vi "CIPT_softwarecontrol with touching pins.vi"() -> ()   [LabVIEW 2022 SP3]
uses:
  Git/CIPT/CIPT/Labview Project/CIPT modes.ctl
  <vilib>/Analysis/baseanly.llb/Mean (DBL).vi
  <vilib>/Utility/file.llb/Read Delimited Spreadsheet (DBL).vi
  <vilib>/Utility/file.llb/Read Delimited Spreadsheet (I64).vi
  <vilib>/gmath/NumericalOptimization/Nonlinear Curve Fit LM.vi
  <vilib>/Utility/file.llb/Write Delimited Spreadsheet (string).vi
  <vilib>/Utility/file.llb/Write Delimited Spreadsheet (I64).vi
  <vilib>/Utility/file.llb/Write Delimited Spreadsheet (DBL).vi
  C:/CIPT/Labview Project/Camera Driver/Labview Driver/OtherDrivers/LabVIEW/ueye.NET/uEyeDotNet.dll
  CIPT/Labview Project/Camera Driver/Labview Driver/OtherDrivers/LabVIEW/ueye.NET/uEyeDotNet.dll
  <vilib>/gmath/NI_Gmath.lvlib
  <instrlib>/Keithley DMM6500 DAQ6500 Series/Keithley DMM6500 DAQ6500 Series.lvlib
  <instrlib>/Keithley 24XX/Keithley 24XX.lvlib
  <instrlib>/Keithley 2182/Keithley 2182.lvlib
  <vilib>/Analysis/NI_AALBase.lvlib
panel:
  out "Array":dbl[](array[numeric])
  out "Comms Errors":errorcluster[](array[cluster])
  in  "Save Filr":bool
  out "error file out":errorcluster
  in  "output file path":path=path "C:/CIPT/Labview Project/csv files/test output.csv"
  in  "stop":bool
  in  "Tab Control":T1(tab)
  in  "Camera ID 3":enum16{"2", "1"}(ring)
  in  "Camera ID 1":enum16{"2", "1"}(ring)
  in  "down a2":bool
  in  "up a2":bool
  in  "down a1":bool
  in  "up a1":bool
  in  "down a3":bool
  in  "up a3":bool
  in  "down all":bool
  in  "up all":bool
  in  "steps /\n continuous \ntoggle":bool
  out "Image first camera":picture
  out "Serial Number 1":string
  in  "Init Camera":bool
  in  "Exit Camera":bool
  in  "Init Camera 2":bool
  in  "Exit Camera 2":bool
  out "Serial Number 2":string
  out "Image second camera":picture
  out "Error Camera 1":errorcluster caption="error"
  out "Error Camera 2":errorcluster caption="error"
  in  "COM 1":refnum<visa-resource-name>
  out "error":errorcluster
  in  "Probe Landing File":path=path "C:/CIPT/Labview Project/csv files/Probe Landing cipt.csv"
  in  "Landing Test on/off?":bool
  in  "load file":bool
  in  "Step size":i32=10
  out "Measurement":sgl[](array[numeric])
  out "Loaded":bool
  out "Loaded":bool
  out "Error Probe Configuration File":errorcluster
  in  "Probe Configuration File":path=path "C:/CIPT/Labview Project/csv files/test probe config.csv"
  in  "Probe Settings File":path=path "C:/CIPT/Labview Project/csv files/deafult_probe_setrings.CSV"
  out "Error Probe Settings File":errorcluster
  out "Probe Spacings":dbl[][](array[numeric])
  in  "Load":bool
  in  "Multiplexer":refnum<visa-resource-name>
  out "all rows":i64[][](array[numeric])
  out "Results Description":string[](array[string])
  out "Results":dbl[][](array[numeric])
  out "Probe Set 2":i32
  in  "Compliance voltage (V)":dbl=42.0
  in  "Measure Instrument":refnum<visa-resource-name>
  in  "Radio Buttons":T2 caption="Select Instrumentation"
  in  "Source Instrument":refnum<visa-resource-name>
  in  "Run":bool
  in  "Current (µA)":dbl=10.0
  out "Measurement Log":string
  out "Probe Set":i32
  in  "Measurement Repeats":i32=10
  in  "Size Of Buffer Used For One Measurement":i32=3
  in  "Top Film R est.":dbl=0.25
  in  "Bottm Film R est.":dbl=0.25
  in  "RA est.":dbl=0.25
  out "Top Film R":dbl
  out "Bottom Film R":dbl
  out "RA":dbl
  out "error out (fitting model)":errorcluster
  in  "Fit Data":bool
  out "Measurements Map Out":map{string, dbl[]}(c390)
  # "Probe Landing cipt_probe check: checks probes individually \nProbe Landing cipt: checks for any connection"
  # "All"
  # "End"
  # "home"
  # "Delete"
  # "Insert"
  # "Page Down"
  # "Page up"
  # "F2"
  # "F1"
  # "Steps"
  # "Continuous"
  # "Probe Settings"
  # "Probe Configuration"
  # "I+"
  # "V+"
  # "V-"
  # "I-"
  # "Max Resolution of 2400 is 300 µV in 200 mV range"
  # "/"
  # "Sheet Resistance (RA)"
  # "Estimated Values"
  # "Fitted Values"
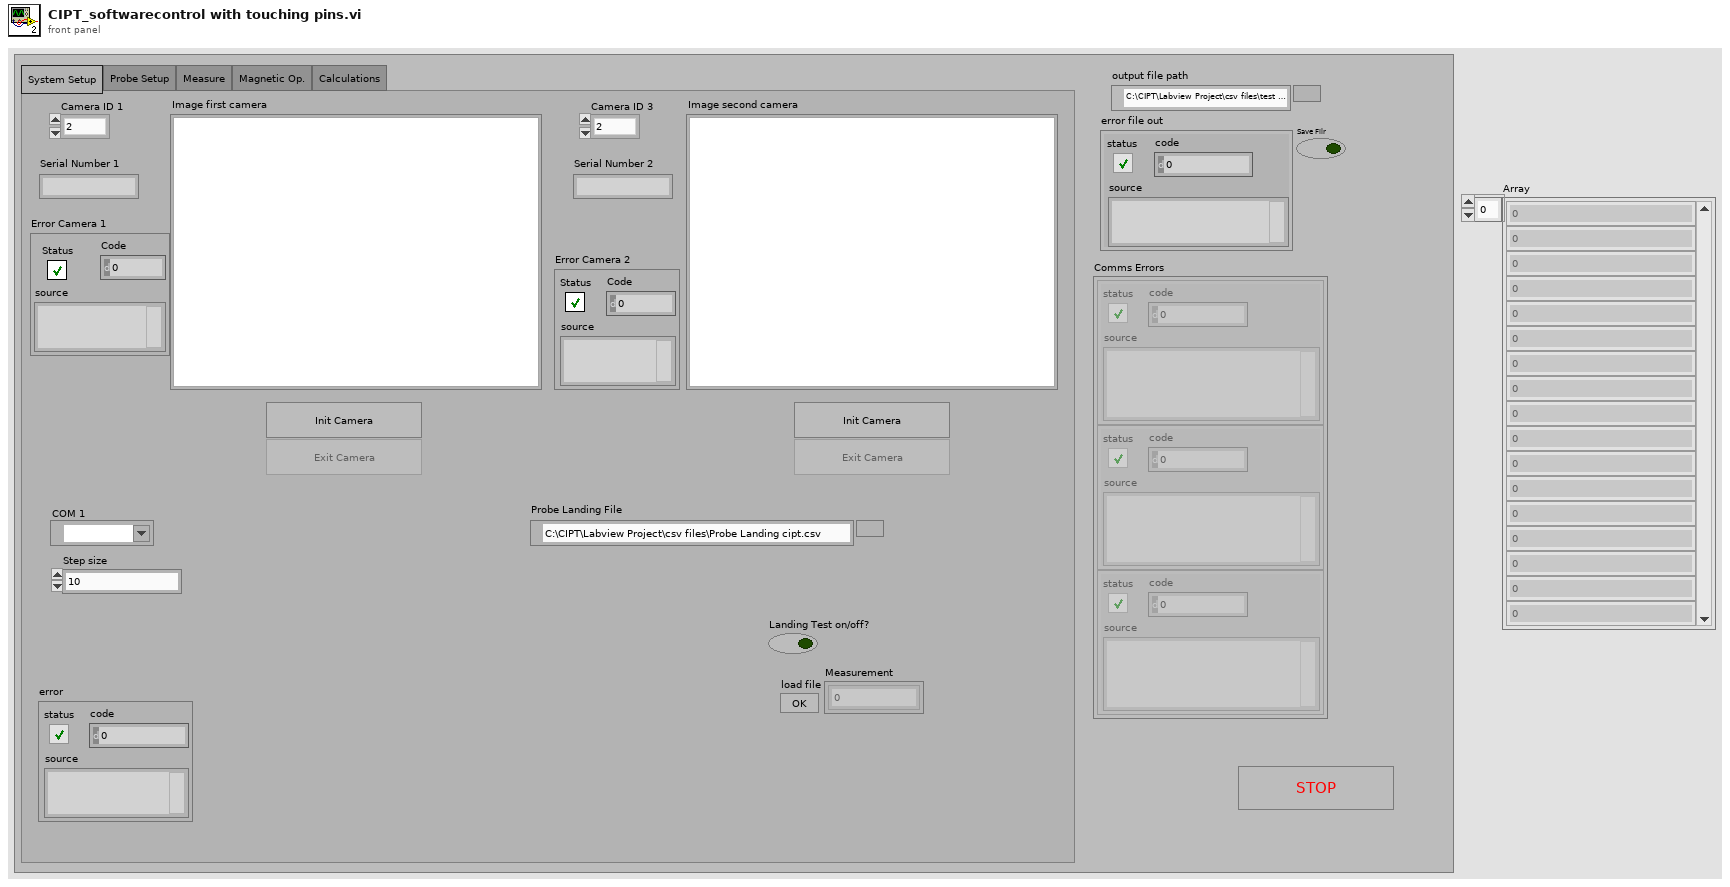
[diagram p1: front panel]
types:
  T1 = enum32{"System Setup", "Probe Setup", "Measure", "Magnetic Op.", "Calculations"}
  T2 = typedef "CIPT modes.ctl" = enum32{"DAQ6510", "2400 Only", "2400 and  2182", "SR830", "SR830 and 6221"}
  T3 = enum32{"System Setup", "Probe Setup", "Measure", "Magnetic Operations", "Calculations + Analyis"}
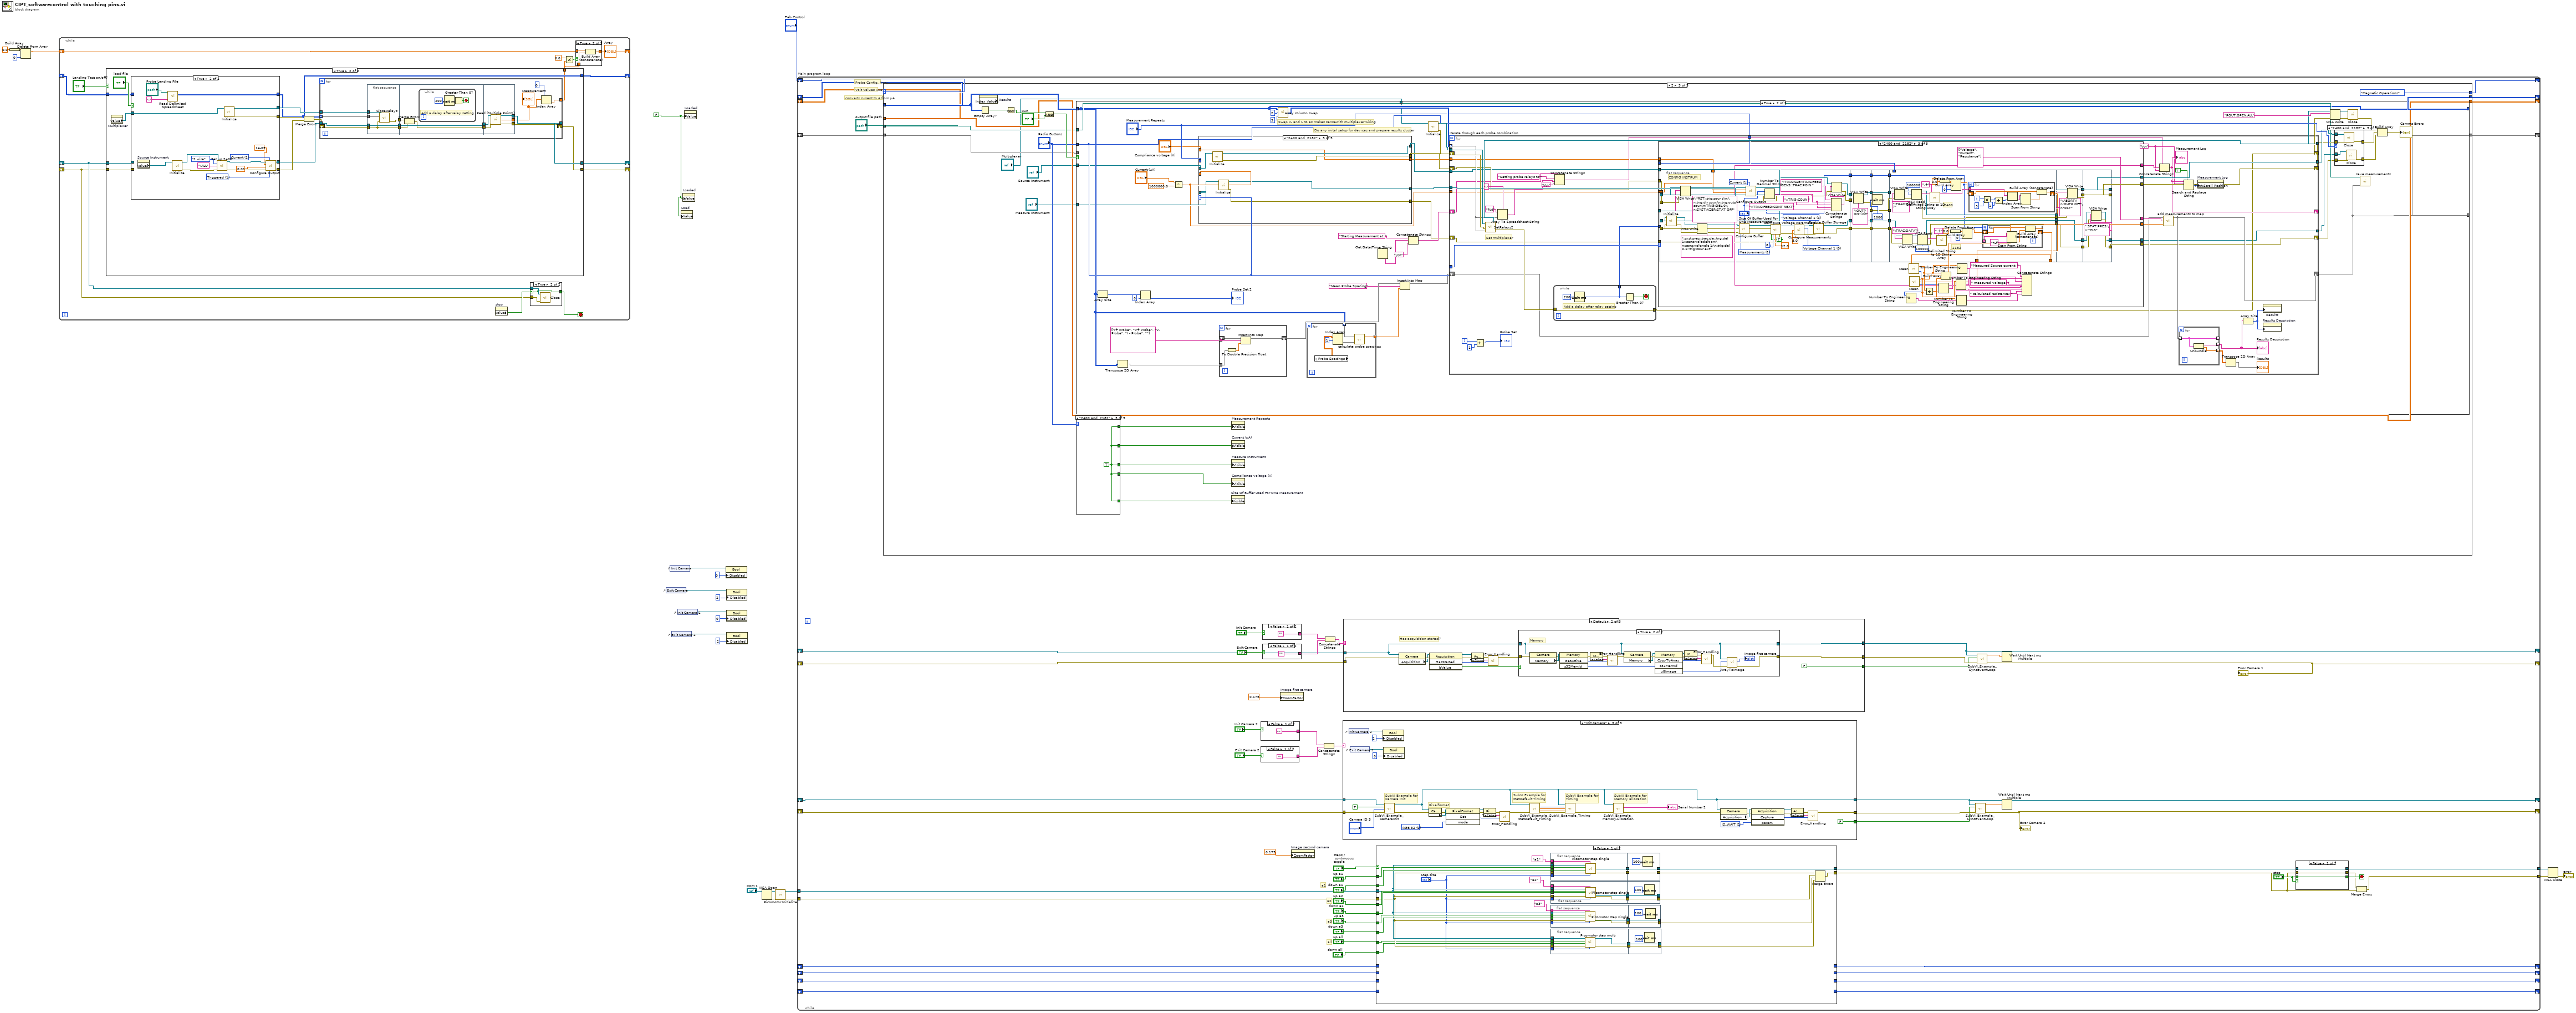
[diagram p0: block diagram]
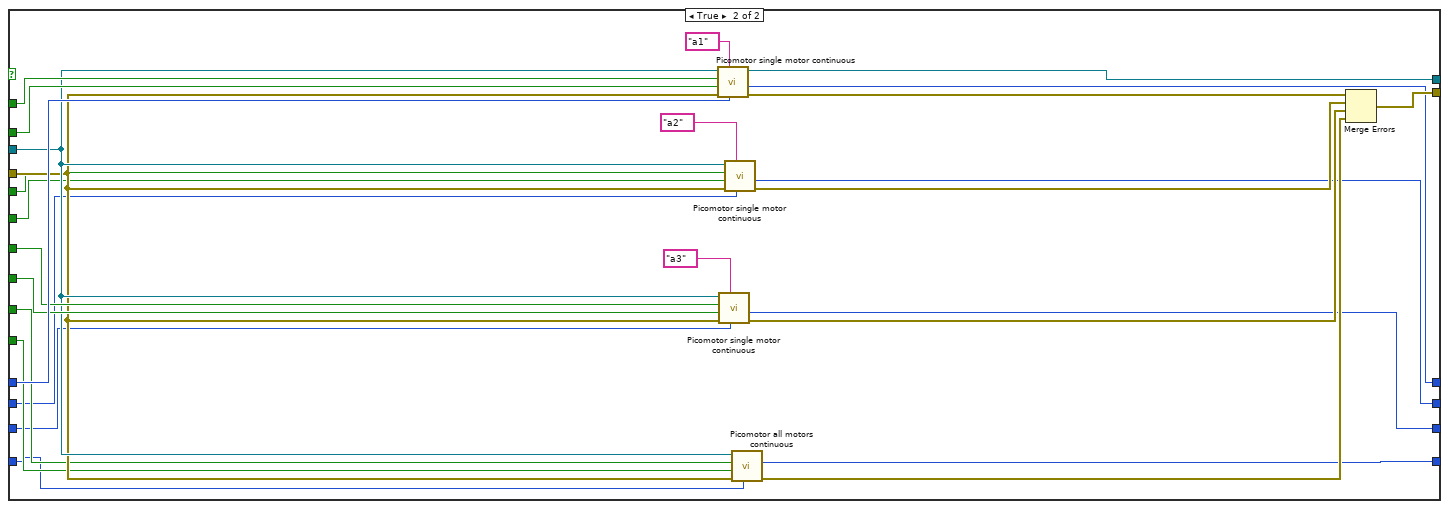
[diagram p6: hidden frame]
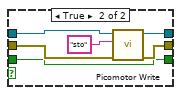
[diagram p7: hidden frame]
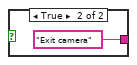
[diagram p8: hidden frame]
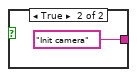
[diagram p9: hidden frame]
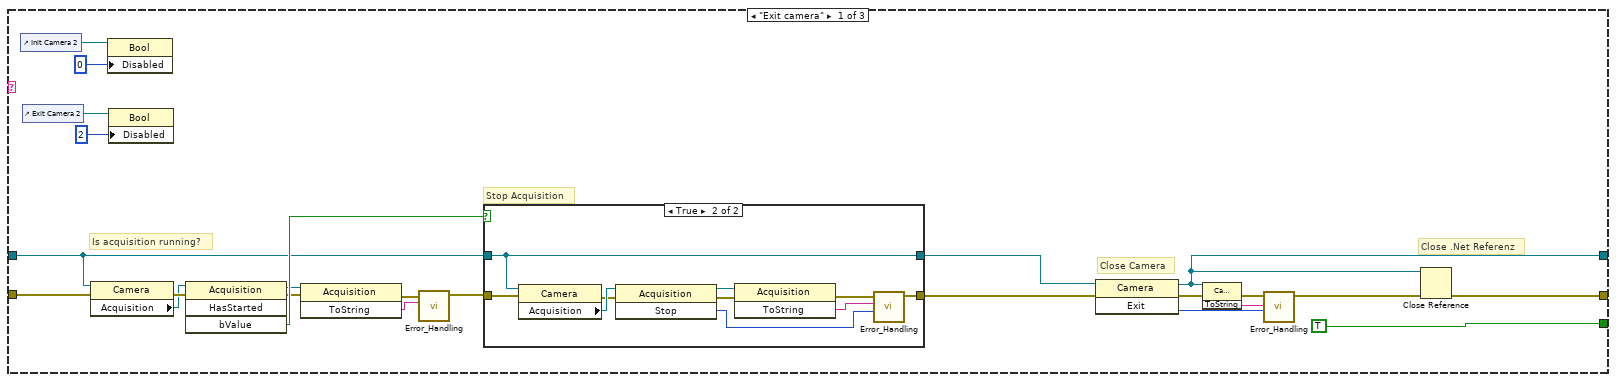
[diagram p10: hidden frame]
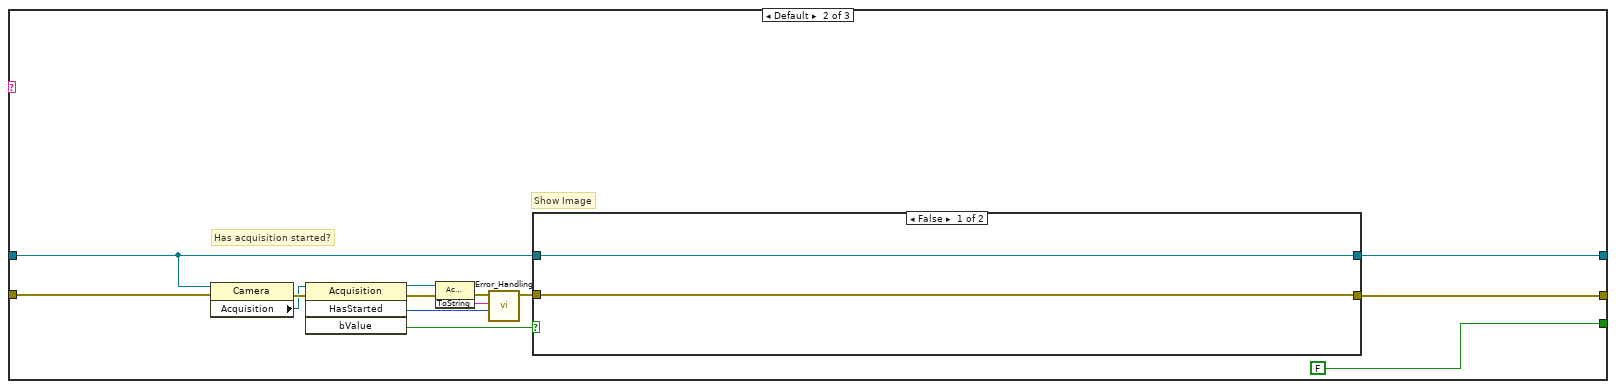
[diagram p12: hidden frame]
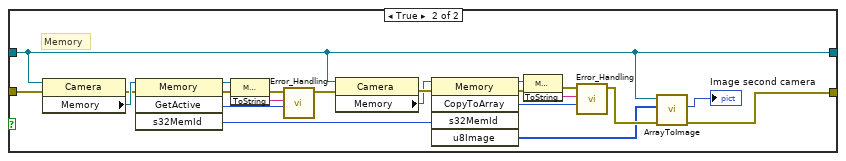
[diagram p13: hidden frame]
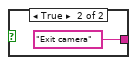
[diagram p14: hidden frame]
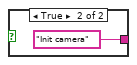
[diagram p15: hidden frame]
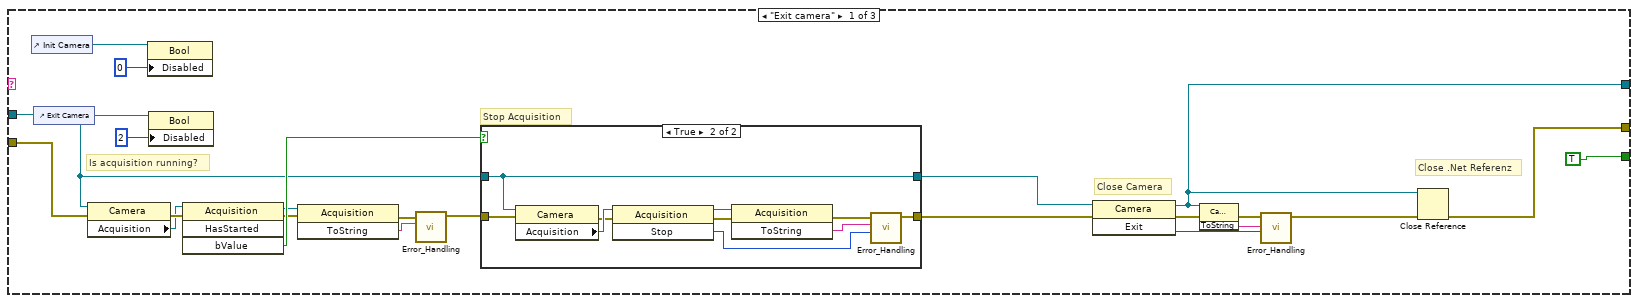
[diagram p16: hidden frame]
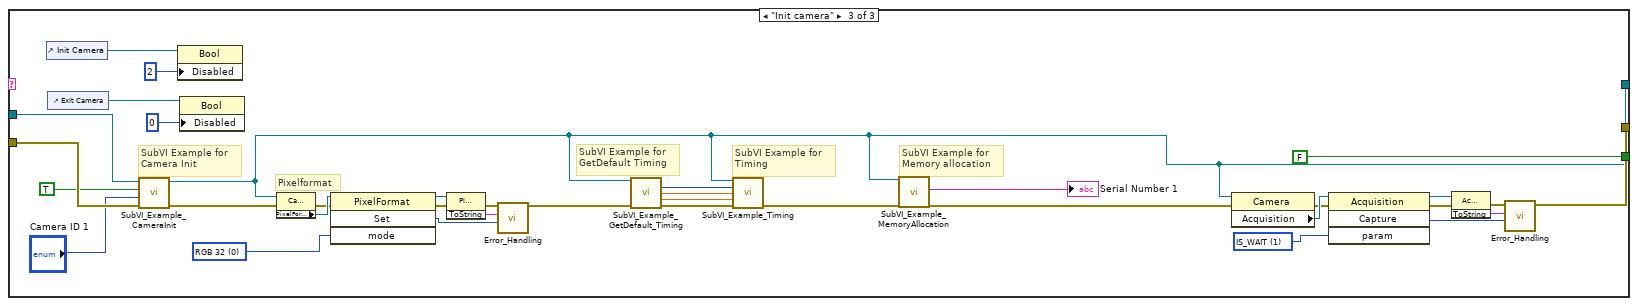
[diagram p19: hidden frame]
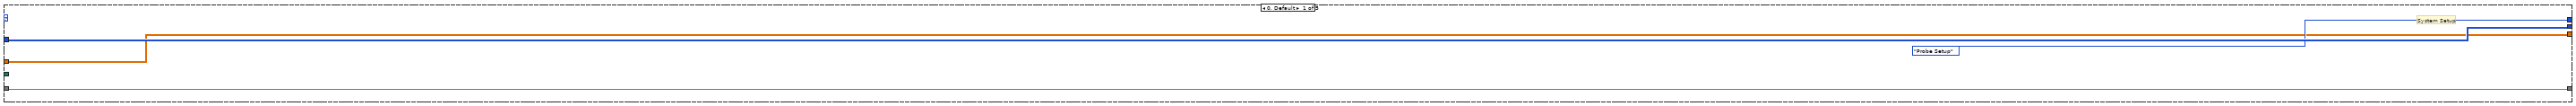
[diagram p20: hidden frame]
diagram:
  w13 = FALSE
  n1 = Build Array(0.0 ("array")) -> (w3:dbl[])
  n2 = Delete From Array(array=w3, index=0) -> (array with subset deleted=w1:dbl[])  [unwired: 1 in, 1 out]
  n3 = while {
    shift-right: [w35] -> _
    shift-left: _ -> [w32]
    shift-right: [w34] -> _
    shift-left: _ -> [w31]
    shift-right: [w29] -> _
    shift-left: _ -> [w28]
    shift-right: [w27] -> _
    shift-left: w1 -> [w26]
    stop <- w30 stop-if-true
    n4 = case shown="True" "Landing Test on/off?" {
      tunnel: w32 -> [w47 w56]
      tunnel: w31 -> [w46 w55]
      tunnel: [w47 w54] -> w35
      tunnel: [w46 w53] -> w34
      tunnel: w28 -> [w45 w50]
      tunnel: [w45 w49] -> w29
      tunnel: [_ w48] -> w24
      frame False {
      }
      frame True {
        n5 = property on="Multiplexer" class="VISAName"() -> ("Value"=w52:refnum<visa-resource-name>)  [unwired: 2 in, 2 out]
        n6 = case shown="True" "load file" {
          tunnel: [_ w99] -> w61
          tunnel: [w95 w102] -> w58
          tunnel: [w96 w101] -> w57
          tunnel: w56 -> [w96 _]
          tunnel: w55 -> [w95 _]
          tunnel: [w94 w100] -> w51
          tunnel: w52 -> [w94 w98]
          tunnel: [w93 w97] -> w49
          tunnel: w50 -> [w93 _]
          frame False {
          }
          frame True {
            w108 = u16 1 items=["Immediate", "Triggered"] ("Output Type  (0: Immediate)")
            w107 = u16 1 items=["Voltage", "Current"] ("Source Mode  (0: Voltage)")
            n7 = property on="Source Instrument" class="VISAName"() -> ("Value"=w113:refnum<visa-resource-name>)  [unwired: 2 in, 2 out]
            n8 = call-poly <vilib>:"Read Delimited Spreadsheet.vi"("file path (dialog if empty)"="Probe Landing File", "delimiter (\\t)"="," ("delimiter (\\t)")) -> ("all rows"=w97:i64[][])  [unwired: 8 in, 5 out]
            n9 = call <instrlib>:"Initialize.vi"("VISA resource name"=w113) -> ("error out"=w110:errorcluster, "VISA resource name out"=w109:refnum<visa-resource-name>)  [unwired: 9 in]
            n10 = call "Set up 2400.vi"("VISA resource name"=w109, "Sense mode"=enum16{"2 wire", "4 wire"}."2 wire", "Measurement Function"=":ALL", "error in (no error)"=w110) -> ("VISA resource name out"=w111:refnum<visa-resource-name>, "error out"=w112:errorcluster)  [unwired: 10 in]
            n11 = call <instrlib>:"Initialize.vi"("VISA resource name"=w98) -> ("error out"=w99:errorcluster, "VISA resource name out"=w100:refnum<visa-resource-name>)  [unwired: 9 in]
            n12 = call <instrlib>:"Configure Output.vi"("Output Type  (0: Immediate)"=w108, "Source Mode  (0: Voltage)"=w107, "error in (no error)"=w112, "Compliance  Level (0.1)"=0.01, "Output Level (0)"=1e-05, "VISA resource name"=w111) -> ("error out"=w102:errorcluster, "VISA resource name out"=w101:refnum<visa-resource-name>)  [unwired: 4 in]
          }
        }
        n13 = Merge Errors(w61, w58) -> (w60:errorcluster)
        n14 = for {
          tunnel: w51 -> [w66]
          shift-right: [w67] -> w53
          shift-left: w60 -> [w70]
          tunnel: w49 -> [w65] mode=indexing
          tunnel: w57 -> [w69]
          tunnel: [w68] -> w54
          tunnel: [w62] -> w48
          n15 = flat-sequence {
            tunnel: w69 -> [w80]
            tunnel: w70 -> [w76]
            tunnel: [w76] -> w75
            tunnel: [w80] -> w74
            tunnel: w66 -> [w79]
            tunnel: [w78] -> w73
            tunnel: w65 -> [w77]
            tunnel: [w82] -> w72
            tunnel: [w84] -> w71
            tunnel: w75 -> [w83]
            tunnel: w74 -> [w84]
            tunnel: w73 -> [w81]
            tunnel: [w90] -> w64
            tunnel: [w89] -> w68
            tunnel: [w88] -> w67
            tunnel: w72 -> [w92]
            tunnel: w71 -> [w91]
            frame #0 {
              n16 = call "CloseRelays.vi"("error in (no error)"=w76, "Array"=w77, "VISA Refnum in"=w79) -> ("error out"=w78:errorcluster)  [unwired: 6 in, 2 out]
            }
            frame #1 {
              n17 = Merge Errors(w81, w83) -> (w82:errorcluster)
              n18 = while {
                stop <- w86 stop-if-true
                # "Add a delay after relay setting"
                n19 = Wait (ms)(milliseconds to wait=u32 200) -> (millisecond timer value=w85:u32)
                n20 = Greater Than 0?(x=w85) -> (x > 0?=w86:bool)
              }
            }
            frame #2 {
              n21 = call <instrlib>:"Read (Multiple Points).vi"("VISA resource name"=w91, "error in (no error)"=w92) -> ("VISA resource name out"=w89:refnum<visa-resource-name>, "Resistance"=w90:sgl[], "error out"=w88:errorcluster)  [unwired: 7 in, 4 out]
            }
          }
          n22 = Index Array(array=w64, index=0) -> (element=w62:sgl)
          "Measurement" <- w64
        }
      }
    }
    n23 = property on="stop" class="Bool (strict)"() -> ("Value"=w33:bool)  [unwired: 2 in, 2 out]
    n24 = case shown="True" w33 {
      selector: w33 -> [w41 w42]
      tunnel: w32 -> [_ w44]
      tunnel: w31 -> [_ w43]
      tunnel: [w41 w42] -> w30
      frame False {
      }
      frame True {
        n25 = call <instrlib>:"Close.vi"("error in (no error)"=w43, "VISA resource name"=w44) -> ()  [unwired: 9 in, 1 out]
      }
    }
    n26 = Not Equal?(x=sgl 0.0, y=w24) -> (x != y?=w25:bool)
    n27 = case shown="True" w25 {
      tunnel: w24 -> [_ w40]
      tunnel: [w37 w39] -> w27
      tunnel: w26 -> [w37 w38]
      frame False {
      }
      frame True {
        n28 = Build Array (concatenate)(w38, w40) -> (w39:dbl[])
      }
    }
    "Array" <- w27
  }
  n29 = control-ref of="Exit Camera"() -> (w16:refnum<vi>)
  n30 = control-ref of="Init Camera"() -> (w17:refnum<vi>)
  n31 = control-ref of="Exit Camera 2"() -> (w21:refnum<vi>)
  n32 = control-ref of="Init Camera 2"() -> (w20:refnum<vi>)
  n33 = property on="Load" class="Bool (strict)"("Value"=w13) -> ()  [unwired: 2 in, 2 out]
  n34 = property on="Loaded" class="Bool (strict)"("Value"=w13) -> ()  [unwired: 2 in, 2 out]
  n35 = property on="Loaded" class="Bool (strict)"("Value"=w13) -> ()  [unwired: 2 in, 2 out]
  n36 = property class="Bool"(reference=w17, "Disabled"=u8 0 ("Deaktiviert")) -> ()  [unwired: 1 in, 2 out]
  n37 = property class="Bool"(reference=w16, "Disabled"=u8 2 ("Deaktiviert")) -> ()  [unwired: 1 in, 2 out]
  n38 = property class="Bool"(reference=w20, "Disabled"=u8 0 ("Deaktiviert")) -> ()  [unwired: 1 in, 2 out]
  n39 = property class="Bool"(reference=w21, "Disabled"=u8 2 ("Deaktiviert")) -> ()  [unwired: 1 in, 2 out]
  n40 = VISA Open(VISA resource name="COM 1") -> (VISA resource name=w11:refnum<visa-resource-name>, error out=w10:errorcluster)  [unwired: 4 in]
  n41 = call "Picomotor Initialize.vi"("error in (no error)"=w10, "VISA Refnum in"=w11) -> ("error out"=w8:errorcluster, "VISA Refnum out"=w9:refnum<visa-resource-name>)  [unwired: 8 in]
  n42 = while "Main program loop" {
    shift-right: [w174] -> _
    shift-left: _ -> [w175]
    shift-right: [w173] -> _
    shift-left: "Tab Control" -> [w176]
    shift-right: [w172] -> _
    shift-left: _ -> [w171]
    shift-right: [w169] -> _
    shift-left: _ -> [w168]
    shift-right: [w157] -> _
    shift-left: _ -> [w155]
    shift-right: [w158] -> _
    shift-left: _ -> [w156]
    shift-right: [w145] -> _
    shift-left: _ -> [w143]
    shift-right: [w144] -> _
    shift-left: _ -> [w142]
    tunnel: w9 -> [w129]
    tunnel: w8 -> [w128]
    tunnel: [w141] -> w6
    shift-right: [w126] -> _
    shift-left: _ -> [w122]
    shift-right: [w125] -> _
    shift-left: _ -> [w121]
    shift-right: [w124] -> _
    shift-left: _ -> [w120]
    shift-right: [w123] -> _
    shift-left: _ -> [w119]
    tunnel: [w116] -> w5
    stop <- w140 stop-if-true
    # "a2"
    # "a3"
    # "all"
    # "a1"
    # "converts current to A from µA"
    # "Volt Values Array"
    # "Probe Config. Array"
    n43 = case shown="2" w176 {
      tunnel: w175 -> [w515 w522 w552 w911 w918]
      tunnel: [w515 w526 w551 w911 w918] -> w174
      tunnel: [T3."Probe Setup" ("Tab Control") T3."Measure" ("Tab Control") T3."Magnetic Operations" ("Tab Control") T3."Calculations + Analyis" ("Tab Control") T3."System Setup" ("Tab Control")] -> w173
      tunnel: [w513 w521 w546 w910 w917] -> w172
      tunnel: w171 -> [w513 w520 w546 w910 w917]
      tunnel: "output file path" -> [_ _ w543 _ w916]
      tunnel: [w512 w517 w542 w909 w915] -> w169
      tunnel: w168 -> [w512 w517 w541 w909 w915]
      frame 0, Default {
        # "System Setup"
      }
      frame 1 {
        # "Probe Setup"
        n44 = Empty Array?(array=w522) -> (empty?=w516:bool)
        n45 = Empty Array?(array=w520) -> (empty?=w519:bool)
        n46 = Not(x=w516) -> (.not. x?=→"Loaded":bool)
        n47 = Not(x=w519) -> (.not. x?=→"Loaded":bool)
        n48 = case shown="True" "Load" {
          tunnel: [w528 w529] -> w526
          tunnel: w522 -> [w528 _]
          tunnel: [w527 w530] -> w521
          tunnel: w520 -> [w527 _]
          frame False {
          }
          frame True {
            # "Probe config. file and data aquisition"
            # "Probe settings file and data aquisition"
            n49 = call-poly <vilib>:"Read Delimited Spreadsheet.vi"("file path (dialog if empty)"="Probe Configuration File", "delimiter (\\t)"="," ("delimiter (\\t)")) -> ("all rows"=w529:i64[][], "error out"=→"Error Probe Configuration File":errorcluster)  [unwired: 8 in, 4 out]
            "all rows" <- w529
            n50 = call-poly <vilib>:"Read Delimited Spreadsheet.vi"("file path (dialog if empty)"="Probe Settings File", "delimiter (\\t)"="," ("delimiter (\\t)")) -> ("all rows"=w530:dbl[][], "error out"=→"Error Probe Settings File":errorcluster)  [unwired: 8 in, 4 out]
            "Probe Spacings" <- w530
          }
        }
        n51 = property on="Load" class="Bool (strict)"("Value"=w516) -> ()  [unwired: 2 in, 2 out]
      }
      frame 2 {
        n52 = property on="Results" class="Arr (strict)" props=["Index Values"]() -> ()  [unwired: 2 in, 3 out]
        n53 = Empty Array?(array=w552) -> (empty?=w554:bool)
        n54 = Not(x=w554) -> (.not. x?=w553:bool)
        n55 = Compound Arithmetic op=AND(w553, "Run") -> (w556:bool)
        n56 = case shown="True" w556 {
          tunnel: w552 -> [w567 w586]
          tunnel: [w567 w586] -> w551
          tunnel: "Radio Buttons" -> [_ w612]
          tunnel: w543 -> [_ w600]
          tunnel: [w566 w582] -> w542
          tunnel: w541 -> [w566 _]
          tunnel: "Measure Instrument" -> [_ w574]
          tunnel: "Source Instrument" -> [_ w573]
          tunnel: "Multiplexer" -> [_ w572]
          frame False {
          }
          frame True {
            # "Swap V- and I- to as makes sensewith multiplexer wiring"
            # "Do any inital setup for devices and prepare results cluster"
            n57 = Array Size(array=w586) -> (size(s)=w606:i32[])
            n58 = Transpose 2D Array(2D array=w586) -> (transposed array=w585:i64[][])
            n59 = Index Array "Index Array"(array=w606, index=0) -> (element=→"Probe Set 2":i32)
            n60 = Divide(x="Current (µA)", y=1000000.0) -> (x/y=w568:dbl)
            n61 = case shown="\"2400 and  2182\"" w612 {
              tunnel: w573 -> [_ w650 w656 _ _]
              tunnel: [_ w638 w655 _ _] -> w613
              tunnel: w574 -> [_ _ w657 _ _]
              tunnel: [_ w638 w653 _ _] -> w576
              tunnel: [_ w644 w652 _ _] -> w607
              tunnel: w568 -> [_ w641 _ _ _]
              tunnel: "Compliance voltage (V)" -> [_ w639 w651 _ _]
              tunnel: "Measurement Repeats" -> [_ _ _ _ _]
              tunnel: [_ _ w654 _ _] -> w571
              tunnel: [_ _ w651 _ _] -> w569
              frame "DAQ6510", Default {
              }
              frame "2400 Only" {
                w642 = u16 1 items=["Immediate", "Triggered"] ("Output Type  (0: Immediate)")
                w643 = u16 1 items=["Voltage", "Current"] ("Source Mode  (0: Voltage)")
                n62 = call <instrlib>:"Initialize.vi"("VISA resource name"=w650) -> ("error out"=w648:errorcluster, "VISA resource name out"=w649:refnum<visa-resource-name>)  [unwired: 9 in]
                n63 = call "Set up 2400.vi"("VISA resource name"=w649, "Sense mode"=enum16{"2 wire", "4 wire"}."4 wire", "Measurement Function"=":ALL", "error in (no error)"=w648) -> ("VISA resource name out"=w646:refnum<visa-resource-name>, "error out"=w645:errorcluster)  [unwired: 10 in]
                n64 = call <instrlib>:"Configure Output.vi"("Output Type  (0: Immediate)"=w642, "Source Mode  (0: Voltage)"=w643, "error in (no error)"=w645, "Compliance  Level (0.1)"=w639, "Output Level (0)"=w641, "VISA resource name"=w646) -> ("error out"=w644:errorcluster, "VISA resource name out"=w638:refnum<visa-resource-name>)  [unwired: 4 in]
              }
              frame "2400 and  2182" {
                n65 = call <instrlib>:"Initialize.vi"("VISA resource name"=w656) -> ("error out"=w652:errorcluster, "VISA resource name out"=w653:refnum<visa-resource-name>)  [unwired: 9 in]
                n66 = call <instrlib>:"Initialize.vi"("VISA resource name"=w657) -> ("error out"=w654:errorcluster, "VISA resource name out"=w655:refnum<visa-resource-name>)  [unwired: 9 in]
              }
              frame "SR830" {
              }
              frame "SR830 and 6221" {
              }
            }
            n67 = for {
              tunnel: w585 -> [w624] mode=indexing
              tunnel: string[] ["I+ Probe", "V+ Probe", "V- Probe", "I - Probe", ""] -> [w625] mode=indexing
              shift-right: [w622] -> w590
              shift-left: _ -> [w621]
              n68 = To Double Precision Float(number=w624) -> (double precision float=w623:dbl[])
              n69 = Insert Into Map(map in=w621, key=w625, value=w623) -> (map out=w622:map{string, dbl[]})  [unwired: 2 out]
            }
            n70 = call "array column swap.vi"("Collumn 2 index"=3, "Collumn 1 index"=2, "Input array"=w586) -> ("output array"=w603:i32[][])
            n71 = for {
              tunnel: w586 -> [w617] mode=indexing
              tunnel: [w616] -> w589 mode=indexing
              n72 = local read "Probe Spacings"() -> (w620:dbl[][])
              n73 = Index Array(array=w620, index (row)=1) -> (element=w618:dbl[])  [unwired: 1 in]
              n74 = call "calculate probe spacings.vi"("Probe Spacings"=w618, "Probe list"=w617) -> ("Mean Spacing"=w616:dbl)  [unwired: 1 out]
            }
            n75 = Get Date/Time String() -> (time string=w609:string)  [unwired: 3 in, 1 out]
            n76 = Insert Into Map(map in=w590, key="Mean Probe Spacing", value=w589) -> (map out=w587:map{string, dbl[]})  [unwired: 2 out]
            n77 = Concatenate Strings("Starting Measurement at: ", w609, "\r\n") -> (w598:string)
            n78 = call <instrlib>:"Initialize.vi"("VISA resource name"=w572) -> ("error out"=w614:errorcluster, "VISA resource name out"=w615:refnum<visa-resource-name>)  [unwired: 9 in]
            n79 = for "Iterate through each probe combination" {
              tunnel: w615 -> [w699]
              tunnel: [w698] -> w596
              tunnel: w603 -> [w692] mode=indexing
              tunnel: w612 -> [w697]
              tunnel: w613 -> [w695]
              shift-right: [w681] -> _
              shift-left: w598 -> [w682]
              shift-right: [w693] -> w610
              shift-left: w607 -> [w686]
              shift-right: [w672] -> w582
              shift-left: w587 -> [w674]
              shift-right: [w666] -> w583
              shift-left: w571 -> [w667]
              tunnel: w576 -> [w685]
              tunnel: [w694] -> w611
              shift-right: [w669] -> w578
              shift-left: w614 -> [w696]
              tunnel: [w665] -> w584
              tunnel: "Measurement Repeats" -> [w664]
              tunnel: w569 -> [w660]
              tunnel: w568 -> [w659]
              i -> [w663]
              w679 = "\r\n"
              # "Set multiplexer"
              n80 = Add(x=w663, y=1) -> (x+y=→"Probe Set":i32)
              n81 = call "SetRelays2.vi"("all rows"=w692, "error in (no error)"=w696, "VISA Refnum in"=w699) -> ("error out"=w687:errorcluster, "VISA resource name out"=w698:refnum<visa-resource-name>)  [unwired: 1 in]
              n82 = Array To Spreadsheet String(delimiter (Tab)=",", array=w692, 3:"%d" ("format string")) -> (spreadsheet string=w688:string)
              n83 = while {
                tunnel: [w706] -> w669
                tunnel: w687 -> [w706]
                tunnel: [w703] -> w668
                stop <- w704 stop-if-true
                # "Add a delay after relay setting"
                n84 = Wait (ms)(milliseconds to wait=u32 200) -> (millisecond timer value=w703:u32)
                n85 = Greater Than 0?(x=w703) -> (x > 0?=w704:bool)
              }
              n86 = Concatenate Strings(w682, "Setting probe relays to:", w688, "\r\n") -> (w677:string)
              n87 = case shown="\"2400 and  2182\"" w697 {
                tunnel: w695 -> [w708 w712 w777 w901 w905]
                tunnel: w685 -> [w707 w733 w785 w902 w906]
                tunnel: w686 -> [w709 w732 w784 w903 w907]
                tunnel: [w707 w730 w745 w902 w906] -> w694
                tunnel: [w709 w729 w753 w903 w907] -> w693
                tunnel: [_ w722 w778 _ _] -> w683
                tunnel: w664 -> [_ w721 w783 _ _]
                tunnel: [_ w715 w782 _ _] -> w675
                tunnel: [_ string[] ["Voltage", "Current", "Resistance"] string[] ["Voltage", "Current", "Resistance"] _ _] -> w676
                tunnel: w668 -> [_ _ _ _ _]
                tunnel: w667 -> [w710 w713 w776 w904 w908]
                tunnel: [w710 w713 w749 w904 w908] -> w666
                tunnel: [w708 w712 w746 w901 w905] -> w665
                tunnel: w660 -> [_ _ w738 _ _]
                tunnel: w659 -> [_ _ w737 _ _]
                frame "DAQ6510", Default {
                }
                frame "2400 Only" {
                  w731 = u16 0 items=["Fixed", "Sweep", "List"] ("Output Mode (0: Fixed)")
                  n88 = call <instrlib>:"Read (Multiple Points).vi"("VISA resource name"=w733, "Sample Count (1)"=w721, "error in (no error)"=w732, "Output Mode (0: Fixed)"=w731) -> ("Voltage"=w711:sgl[], "VISA resource name out"=w730:refnum<visa-resource-name>, "Current"=w720:sgl[], "Resistance"=w719:sgl[], "error out"=w729:errorcluster)  [unwired: 5 in, 2 out]
                  n89 = call-poly <vilib>:"Mean.vi"("X"=w711) -> ("mean"=w718:dbl)  [unwired: 1 out]
                  n90 = call-poly <vilib>:"Mean.vi"("X"=w720) -> ("mean"=w717:dbl)  [unwired: 1 out]
                  n91 = call-poly <vilib>:"Mean.vi"("X"=w719) -> ("mean"=w716:dbl)  [unwired: 1 out]
                  n92 = Build Array(w718, w717, w716) -> (w715:dbl[])
                  n93 = Number To Engineering String(4:w718) -> (0:w723:string)  [unwired: 3 in]
                  n94 = Number To Engineering String(4:w717) -> (0:w727:string)  [unwired: 3 in]
                  n95 = Number To Engineering String(4:w716) -> (0:w724:string)  [unwired: 3 in]
                  n96 = Concatenate Strings("Measured I = ", w727, " V = " ("string"), w723, "R = " ("string"), w724) -> (w722:string)
                }
                frame "2400 and  2182" {
                  n97 = flat-sequence {
                    tunnel: w776 -> [w792]
                    tunnel: w777 -> [w793]
                    tunnel: w784 -> [w794]
                    tunnel: w785 -> [w795]
                    tunnel: [w799] -> w748
                    tunnel: [w798] -> w747
                    tunnel: [w797] -> w740
                    tunnel: [w796] -> w739
                    tunnel: w738 -> [w790]
                    tunnel: w737 -> [w789]
                    tunnel: ["Size Of Buffer Used For One Measurement"] -> w734
                    tunnel: [w832] -> w765
                    tunnel: [w831] -> w763
                    tunnel: [w829] -> w760
                    tunnel: [w828] -> w758
                    tunnel: w748 -> [w832]
                    tunnel: w747 -> [w831]
                    tunnel: w740 -> [w830]
                    tunnel: w739 -> [_]
                    tunnel: [w826] -> w735
                    tunnel: w734 -> [w826]
                    tunnel: w765 -> [w838]
                    tunnel: [w838] -> w764
                    tunnel: w763 -> [w837]
                    tunnel: [w837] -> w762
                    tunnel: [w835] -> w761
                    tunnel: w760 -> [w835]
                    tunnel: [w834] -> w759
                    tunnel: w758 -> [w834]
                    tunnel: [w833] -> w736
                    tunnel: w735 -> [w833]
                    tunnel: w783 -> [_]
                    tunnel: w764 -> [w848]
                    tunnel: w762 -> [w847]
                    tunnel: w761 -> [w850]
                    tunnel: w759 -> [w849]
                    tunnel: [w846] -> w757
                    tunnel: [w845] -> w756
                    tunnel: [w843] -> w755
                    tunnel: [w842] -> w754
                    tunnel: [w841] -> w751
                    tunnel: [w840] -> w750
                    tunnel: w736 -> [w839]
                    tunnel: w755 -> [w893]
                    tunnel: w754 -> [w892]
                    tunnel: w751 -> [w888]
                    tunnel: w750 -> [w889]
                    tunnel: [w890] -> w744
                    tunnel: [w889] -> w743
                    tunnel: [w888] -> w742
                    tunnel: [w887] -> w741
                    tunnel: [w899] -> w745
                    tunnel: [w894] -> w746
                    tunnel: [w895] -> w749
                    tunnel: [w900] -> w753
                    tunnel: w744 -> [w900]
                    tunnel: w743 -> [w896]
                    tunnel: w742 -> [w897]
                    tunnel: w741 -> [w899]
                    frame #0 {
                      w803 = 0 items=["Voltage Channel 1", "Voltage Channel 2", "Temperature Channel 1", "Temperature Channel 2"] ("Measurement (0: Voltage Channel 1)")
                      w791 = u16 1 items=["Voltage", "Current"] ("Source Mode  (0: Voltage)")
                      w816 = 1 items=["Voltage Channel 1"=1, "Voltage Channel 2"=2] ("Measurement (1: Voltage Channel 1)")
                      w817 = 1 items=["None", "Measurements", "Math Calculation"] ("Buffer Source (0: None)")
                      # "CONFIG INSTRUM"
                      n98 = call <instrlib>:"Initialize.vi"("error in (no error)"=w792, "VISA resource name"=w793) -> ("error out"=w801:errorcluster, "VISA resource name out"=w802:refnum<visa-resource-name>)  [unwired: 8 in]
                      n99 = VISA Write(VISA resource name=w795, write buffer=":*RST;:trig:sour tlin;\n:trig:dir sour;\n:trig:outp sour;\n:TRIG:DEL 0;\n:SYST:AZER:STAT OFF", error in (no error)=w794) -> (VISA resource name out=w812:refnum<visa-resource-name>, error out=w807:errorcluster)  [unwired: 1 out]
                      n100 = VISA Write(VISA resource name=w802, write buffer=":syst:pres;:trac:cle;:trig:del 1;:sens:volt:delt on;\n:sens:volt:nplc 1;\n:trig:del 0.1;:trig:sour ext", error in (no error)=w801) -> (VISA resource name out=w814:refnum<visa-resource-name>, error out=w813:errorcluster)  [unwired: 1 out]
                      n101 = call <instrlib>:"Configure Buffer.vi"("error in (no error)"=w813, "Buffer Source (0: None)"=w817, "Buffer Size (2)"="Size Of Buffer Used For One Measurement", "VISA resource name"=w814) -> ("error out"=w818:errorcluster, "VISA resource name out"=w821:refnum<visa-resource-name>)  [unwired: 6 in]
                      n102 = call <instrlib>:"Configure Output.vi"("Source Mode  (0: Voltage)"=w791, "error in (no error)"=w807, "Compliance  Level (0.1)"=w790, "Output Level (0)"=w789, "VISA resource name"=w812) -> ("error out"=w806:errorcluster, "VISA resource name out"=w788:refnum<visa-resource-name>)  [unwired: 5 in]
                      n103 = Number To Decimal String(number="Size Of Buffer Used For One Measurement") -> (decimal integer string=w808:string)  [unwired: 1 in]
                      n104 = call <instrlib>:"Configure Voltage Parameters.vi"("VISA resource name"=w821, "Measurement (1: Voltage Channel 1)"=w816, "Voltage Resolution (8)"=8, "Range Value (12)"=12.0, "Autorange (T: Enable)"=TRUE, "error in (no error)"=w818) -> ("VISA resource name out"=w820:refnum<visa-resource-name>, "error out"=w819:errorcluster)  [unwired: 8 in]
                      n105 = call <instrlib>:"Configure Measurements.vi"("VISA resource name"=w820, "Measurement (0: Voltage Channel 1)"=w803, "Integration Rate (5)"=5.0, "error in (no error)"=w819) -> ("VISA resource name out"=w805:refnum<visa-resource-name>, "error out"=w804:errorcluster)  [unwired: 10 in]
                      n106 = call <instrlib>:"Enable Buffer Storage.vi"("error in (no error)"=w804, "VISA resource name"=w805) -> ("error out"=w798:errorcluster, "VISA resource name out"=w799:refnum<visa-resource-name>)  [unwired: 8 in]
                      n107 = Concatenate Strings(":TRAC:CLE;:TRAC:FEED SENS;:TRAC:POIN " ("write buffer"), w808, ";:TRIG:COUN " ("write buffer"), w808, ";:TRAC:FEED:CONT NEXT" ("write buffer")) -> (w787:string)
                      n108 = VISA Write(VISA resource name=w788, write buffer=w787, error in (no error)=w806) -> (VISA resource name out=w797:refnum<visa-resource-name>, error out=w796:errorcluster)  [unwired: 1 out]
                    }
                    frame #1 {
                      n109 = VISA Write(VISA resource name=w830, write buffer=":OUTP ON;:init") -> (VISA resource name out=w829:refnum<visa-resource-name>, error out=w828:errorcluster)  [unwired: 1 in, 1 out]
                    }
                    frame #2 {
                      n110 = Wait (ms)(milliseconds to wait=u32 1000) -> ()  [unwired: 1 out]
                    }
                    frame #3 {
                      # "2182"
                      # "2400"
                      n111 = VISA Write(VISA resource name=w850, write buffer=":TRAC:DATA?", error in (no error)=w849) -> (VISA resource name out=w860:refnum<visa-resource-name>, error out=w859:errorcluster)  [unwired: 1 out]
                      n112 = VISA Write(VISA resource name=w848, write buffer=":TRAC:DATA?", error in (no error)=w847) -> (VISA resource name out=w869:refnum<visa-resource-name>, error out=w868:errorcluster)  [unwired: 1 out]
                      n113 = VISA Read(VISA resource name=w860, byte count=u32 100000, error in (no error)=w859) -> (VISA resource name out=w843:refnum<visa-resource-name>, read buffer=w856:string, error out=w842:errorcluster)  [unwired: 1 out]
                      n114 = VISA Read(VISA resource name=w869, byte count=u32 100000, error in (no error)=w868) -> (VISA resource name out=w841:refnum<visa-resource-name>, read buffer=w866:string, error out=w840:errorcluster)  [unwired: 1 out]
                      n115 = call <vilib>:"Delimited String to 1D String Array.vi"("delimiter"=",+" ("delimiter (Tab)"), "delimited string"=w856) -> ("string array"=w852:string[])  [unwired: 9 in]
                      n116 = call <vilib>:"Delimited String to 1D String Array.vi"("delimiter"=",+" ("delimiter (Tab)"), "delimited string"=w866) -> ("string array"=w861:string[])  [unwired: 9 in]
                      n117 = Build Array(0.0 ("array")) -> (w854:dbl[])
                      n118 = Build Array(0.0 ("array")) -> (w864:dbl[])
                      n119 = Delete From Array(array=w854, index=0) -> (array with subset deleted=w844:dbl[])  [unwired: 1 in, 1 out]
                      n120 = Delete From Array(array=w864, index=0) -> (array with subset deleted=w862:dbl[])  [unwired: 1 in, 1 out]
                      n121 = for {
                        N: w839 -> [_]
                        shift-right: [w875] -> w845
                        shift-left: w844 -> [w874]
                        tunnel: w852 -> [w873]
                        i -> [w881]
                        n122 = Multiply(x=w881, y=5) -> (x*y=w880:i32)
                        n123 = Add(x=w880, y=1) -> (x+y=w877:i32)
                        n124 = Index Array(array=w873, index=w877) -> (element=w872:string)
                        n125 = Scan From String(input string=w872) -> (output 1=w876:dbl)  [unwired: 4 in, 3 out]
                        n126 = Build Array (concatenate)(w874, w876) -> (w875:dbl[])
                      }
                      n127 = for {
                        N: w839 -> [_]
                        shift-right: [w884] -> w846
                        shift-left: w862 -> [w883]
                        tunnel: w861 -> [w882] mode=indexing
                        n128 = Scan From String(format string="%f", input string=w882) -> (output 1=w885:dbl)  [unwired: 3 in, 3 out]
                        n129 = Build Array (concatenate)(w883, w885) -> (w884:dbl[])
                      }
                    }
                    frame #4 {
                      n130 = VISA Write(VISA resource name=w893, write buffer=":ABORT;\n:OUTP OFF;\n*RST" ("data"), error in (no error)=w892) -> (VISA resource name out=w887:refnum<visa-resource-name>, error out=w890:errorcluster)  [unwired: 1 out]
                    }
                    frame #5 {
                      n131 = VISA Write(VISA resource name=w897, write buffer=":STAT:PRES;\n:*CLS" ("data"), error in (no error)=w896) -> (VISA resource name out=w894:refnum<visa-resource-name>, error out=w895:errorcluster)  [unwired: 1 out]
                    }
                  }
                  n132 = call-poly <vilib>:"Mean.vi"("X"=w757) -> ("mean"=w781:dbl, "error"=w769:i32)
                  n133 = Number To Engineering String(4:w769) -> (0:w768:string)  [unwired: 3 in]
                  n134 = call-poly <vilib>:"Mean.vi"("X"=w756) -> ("mean"=w780:dbl, "error"=w773:i32)
                  n135 = Divide(x=w781, y=w780) -> (x/y=w779:dbl)
                  n136 = Number To Engineering String(4:w773) -> (0:w772:string)  [unwired: 3 in]
                  n137 = Build Array(w781, w780, w779) -> (w782:dbl[])
                  n138 = Number To Engineering String(4:w780) -> (0:w774:string)  [unwired: 3 in]
                  n139 = Number To Engineering String(4:w779) -> (0:w766:string)  [unwired: 3 in]
                  n140 = Number To Engineering String(4:w781) -> (0:w770:string)  [unwired: 3 in]
                  n141 = Concatenate Strings("Measured Source current: " ("string"), w774, w772, " measured voltage: " ("string"), w770, w768, " calculated resistance: " ("string"), w766) -> (w778:string)
                }
                frame "SR830" {
                }
                frame "SR830 and 6221" {
                }
              }
              n142 = Concatenate Strings(w677, w683, w679) -> (w681:string)
              "Measurement Log" <- w681
              n143 = call "add measurements to map.vi"("Measurement Values"=w675, "Measurement Names"=w676, "Measurements Map in"=w674) -> ("Measurements Map Out"=w672:map{string, dbl[]})  [unwired: 2 in]
              n144 = for {
                tunnel: [w702] -> _ mode=indexing
                tunnel: w672 -> [w702] mode=indexing
                tunnel: [w701] -> w671 mode=indexing
                tunnel: [w700] -> w670 mode=indexing
                n145 = Unbundle(w702) -> (w701:string, "Array"=w700:dbl[])
              }
              "Results Description" <- w671
              n146 = Search and Replace String(replace all?=TRUE, input string=w681, search string=w679) -> (number of replacements=w678:i32)  [unwired: 5 in, 3 out]
              n147 = property on="Measurement Log" class="Str"("Text.Scroll Position"=w678) -> ()  [unwired: 2 in, 2 out]
              n148 = Transpose 2D Array(2D array=w670) -> (transposed array=→"Results":dbl[][])
              n149 = Array Size(array=w671) -> (size(s)=w673:i32)
              n150 = property on="Results" class="Arr (strict)"("Number of Columns"=w673) -> ()  [unwired: 2 in, 2 out]
              n151 = property on="Results Description" class="Arr (strict)"("Number of Columns"=w673) -> ()  [unwired: 2 in, 2 out]
            }
            n152 = VISA Write(VISA resource name=w596, write buffer="ROUT:OPEN:ALL", error in (no error)=w578) -> (VISA resource name out=w595:refnum<visa-resource-name>, error out=w594:errorcluster)  [unwired: 1 out]
            n153 = case shown="\"2400 and  2182\"" w612 {
              tunnel: w611 -> [_ w631 w636 _ _]
              tunnel: w610 -> [w627 w630 w637 _ _]
              tunnel: [w627 w629 w632 _ _] -> w581
              tunnel: w584 -> [_ _ w635 _ _]
              tunnel: w583 -> [w626 w628 w634 _ _]
              tunnel: [w626 w628 w633 _ _] -> w580
              frame "DAQ6510", Default {
              }
              frame "2400 Only" {
                n154 = call <instrlib>:"Close.vi"("error in (no error)"=w630, "VISA resource name"=w631) -> ("error out"=w629:errorcluster)  [unwired: 9 in]
              }
              frame "2400 and  2182" {
                n155 = call <instrlib>:"Close.vi"("error in (no error)"=w637, "VISA resource name"=w636) -> ("error out"=w632:errorcluster)  [unwired: 9 in]
                n156 = call <instrlib>:"Close.vi"("error in (no error)"=w634, "VISA resource name"=w635) -> ("error out"=w633:errorcluster)  [unwired: 9 in]
              }
              frame "SR830" {
              }
              frame "SR830 and 6221" {
              }
            }
            n157 = call <instrlib>:"Close.vi"("error in (no error)"=w594, "VISA resource name"=w595) -> ("error out"=w577:errorcluster)  [unwired: 9 in]
            n158 = call "save measurements.vi"("Save path"=w600, "Measurements In"=w582) -> ()  [unwired: 12 in, 2 out]
            n159 = Build Array(w577, w581, w580) -> (→"Comms Errors":errorcluster[])
          }
        }
        n160 = case shown="\"2400 and  2182\"" "Radio Buttons" {
          tunnel: [w557 w559 w561 w562 w565] -> w550
          tunnel: [w557 w560 w561 w562 w564] -> w549
          tunnel: [TRUE w560 w561 TRUE w565] -> w545
          tunnel: [w557 w560 w561 w562 w565] -> w544
          tunnel: [w557 w559 w561 w562 w564] -> w537
          frame "DAQ6510", Default {
            w557 = FALSE
          }
          frame "2400 Only" {
            w560 = TRUE
            w559 = FALSE
          }
          frame "2400 and  2182" {
            w561 = TRUE
          }
          frame "SR830" {
            w562 = FALSE
          }
          frame "SR830 and 6221" {
            w564 = FALSE
            w565 = TRUE
          }
        }
        n161 = property on="Size Of Buffer Used For One Measurement" class="DigNum (strict)"("Visible"=w537) -> ()  [unwired: 2 in, 2 out]
        n162 = property on="Measurement Repeats" class="DigNum (strict)"("Visible"=w545) -> ()  [unwired: 2 in, 2 out]
        n163 = property on="Current (µA)" class="DigNum (strict)"("Visible"=w549) -> ()  [unwired: 2 in, 2 out]
        n164 = property on="Measure Instrument" class="VISAName"("Visible"=w550) -> ()  [unwired: 2 in, 2 out]
        n165 = property on="Compliance voltage (V)" class="DigNum (strict)"("Visible"=w544) -> ()  [unwired: 2 in, 2 out]
      }
      frame 3 {
        # "Magnetic Op."
      }
      frame 4 {
        # "Calculations"
        # "Save File - saves collected data into a (csv) file and asks for a file path if not already given"
        n166 = Look In Map(map=w915, key="Resistance") -> (value=w913:dbl[])  [unwired: 1 in, 1 out]
        n167 = Build Array("Top Film R est.", "Bottm Film R est.", "RA est.") -> (w923:dbl[])
        n168 = case shown="True" "Fit Data" {
          tunnel: w918 -> [_ w943]
          tunnel: w923 -> [_ w941]
          tunnel: [dbl[] [0.0, 0.0, 0.0] w932] -> w920
          tunnel: w913 -> [_ w930]
          frame False {
          }
          frame True {
            # "Calculated R"
            # "Mean probe spacing"
            n169 = Index Array(array=w943, index (col)=4 ("disabled index (col)")) -> (element=w942:i64[])  [unwired: 1 in]
            n170 = vi-ref "modelFunction.vi"() -> (w940:refnum<vi>)
            n171 = call-poly <vilib>:"Nonlinear Curve Fit.vi"("Y"=w930, "f(x,a)"=w940, "X"=w942, "initial parameters"=w941) -> ("best fit parameters"=w932:dbl[], "error out"=→"error out (fitting model)":errorcluster)  [unwired: 6 in, 4 out]
            n172 = Index Array(array=w932, index=0) -> (element=→"Top Film R":dbl)
            n173 = Index Array(array=w932, index=1) -> (element=→"Bottom Film R":dbl)
            n174 = Index Array(array=w932, index=2) -> (element=→"RA":dbl)
          }
        }
        n175 = case shown="True" "Save Filr" {
          tunnel: w918 -> [_ w964]
          tunnel: string[] ["I+", "V+", "V-", "I-", "x (mean probe spacing)", "V", "I (µA)", "R (=V/I)"] -> [_ w960]
          tunnel: string[] ["R (t)", "R (b)", "RA"] -> [_ w952]
          tunnel: w920 -> [_ w945]
          tunnel: w916 -> [_ w944]
          frame False {
          }
          frame True {
            n176 = call-poly <vilib>:"Write Delimited Spreadsheet.vi"("file path (dialog if empty)"=w944, "1D data"=w960, "delimiter (\\t)"="," ("delimiter (\\t)")) -> ("new file path (Not A Path if cancelled)"=w962:path, "error out"=w961:errorcluster)  [unwired: 11 in]
            n177 = call-poly <vilib>:"Write Delimited Spreadsheet.vi"("file path (dialog if empty)"=w962, "format (%d)"="%.6f" ("format (%.3f)"), "2D data"=w964, "append to file? (new file:F)"=TRUE, "error in (no error)"=w961, "delimiter (\\t)"="," ("delimiter (\\t)")) -> ("new file path (Not A Path if cancelled)"=w954:path, "error out"=w953:errorcluster)  [unwired: 8 in]
            n178 = call-poly <vilib>:"Write Delimited Spreadsheet.vi"("file path (dialog if empty)"=w954, "format (%s)"="%.6f" ("format (%.3f)"), "1D data"=w952, "append to file? (new file:F)"=TRUE, "error in (no error)"=w953, "delimiter (\\t)"="," ("delimiter (\\t)")) -> ("new file path (Not A Path if cancelled)"=w947:path, "error out"=w946:errorcluster)  [unwired: 8 in]
            n179 = call-poly <vilib>:"Write Delimited Spreadsheet.vi"("file path (dialog if empty)"=w947, "format (%.3f)"="%.6f", "1D data"=w945, "append to file? (new file:F)"=TRUE, "error in (no error)"=w946, "delimiter (\\t)"="," ("delimiter (\\t)")) -> ("error out"=→"error file out":errorcluster)  [unwired: 8 in, 1 out]
          }
        }
        "Measurements Map Out" <- w915
      }
    }
    n180 = case shown="False" "Exit Camera 2" {
      tunnel: ["" "Exit camera"] -> w150
      frame False {
      }
      frame True {
      }
    }
    n181 = case shown="False" "Init Camera 2" {
      tunnel: ["" "Init camera"] -> w153
      frame False {
      }
      frame True {
      }
    }
    n182 = case shown="False" "Init Camera" {
      tunnel: ["" "Init camera"] -> w166
      frame False {
      }
      frame True {
      }
    }
    n183 = case shown="False" "Exit Camera" {
      tunnel: ["" "Exit camera"] -> w163
      frame False {
      }
      frame True {
      }
    }
    n184 = property on="Image first camera" class="Pict"("ZoomFactor"=0.175) -> ()  [unwired: 2 in, 2 out]
    n185 = property on="Image second camera" class="Pict"("ZoomFactor"=0.175) -> ()  [unwired: 2 in, 2 out]
    n186 = Concatenate Strings(w153, w150) -> (w152:string)
    n187 = Concatenate Strings(w166, w163) -> (w165:string)
    n188 = case shown="\"Init camera\"" w152 {
      tunnel: w143 -> [w294 w325 w390]
      tunnel: w142 -> [w295 w324 w389]
      tunnel: [w304 w327 w368] -> w145
      tunnel: [w305 w326 w369] -> w149
      tunnel: [TRUE FALSE FALSE] -> w147
      frame "Exit camera" {
        # "Close .Net Referenz"
        # "Is acquisition running?"
        # "Stop Acquisition"
        # "Close Camera"
        n189 = control-ref of="Init Camera 2"() -> (w289:refnum<vi>)
        n190 = control-ref of="Exit Camera 2"() -> (w288:refnum<vi>)
        n191 = property class="Camera"(reference=w294, error in=w295) -> (error out=w303:errorcluster, "Acquisition"=w302:refnum<k24>)  [unwired: 1 out]
        n192 = property class="Bool"(reference=w289, "Disabled"=u8 0 ("Deaktiviert")) -> ()  [unwired: 1 in, 2 out]
        n193 = property class="Bool"(reference=w288, "Disabled"=u8 2 ("Deaktiviert")) -> ()  [unwired: 1 in, 2 out]
        n194 = invoke class="Acquisition" method="HasStarted"(reference=w302, error in=w303) -> (reference out=w296:refnum<k24>, error out=w299:errorcluster, "bValue"=w301:bool)  [unwired: 2 in, 1 out]
        n195 = invoke class="Acquisition" method="ToString"(reference=w296, error in=w299) -> (error out=w298:errorcluster, "ToString"=w297:string)  [unwired: 1 in, 1 out]
        n196 = call <instrlib>:"Error_Handling.vi"("Error String"=w297, "Error In"=w298) -> ("Error Out"=w300:errorcluster)  [unwired: 9 in]
        n197 = case shown="True" w301 {
          tunnel: [w313 w322] -> w292
          tunnel: w300 -> [w313 w323]
          tunnel: w294 -> [w312 w314]
          tunnel: [w312 w314] -> w293
          frame False {
          }
          frame True {
            n198 = property class="Camera"(reference=w314, error in=w323) -> (error out=w318:errorcluster, "Acquisition"=w319:refnum<k24>)  [unwired: 1 out]
            n199 = invoke class="Acquisition" method="Stop"(reference=w319, error in=w318) -> (reference out=w316:refnum<k24>, error out=w317:errorcluster, "Stop"=w315:i32)  [unwired: 1 in]
            n200 = invoke class="Acquisition" method="ToString"(reference=w316, error in=w317) -> (error out=w321:errorcluster, "ToString"=w320:string)  [unwired: 1 in, 1 out]
            n201 = call <instrlib>:"Error_Handling.vi"("Error Code"=w315, "Error String"=w320, "Error In"=w321) -> ("Error Out"=w322:errorcluster)  [unwired: 8 in]
          }
        }
        n202 = invoke class="Camera" method="Exit"(reference=w293, error in=w292) -> (reference out=w304:refnum<k24>, error out=w308:errorcluster, "Exit"=w307:i32)  [unwired: 1 in]
        n203 = invoke class="Camera" method="ToString"(reference=w304, error in=w308) -> (error out=w309:errorcluster, "ToString"=w310:string)  [unwired: 1 in, 1 out]
        n204 = call <instrlib>:"Error_Handling.vi"("Error Code"=w307, "Error String"=w310, "Error In"=w309) -> ("Error Out"=w306:errorcluster)  [unwired: 8 in]
        n205 = Close Reference ("Close Referenz")(reference=w304, error in (no error)=w306) -> (error out=w305:errorcluster)
      }
      frame Default {
        # "Has acquisition started?"
        # "Show Image"
        n206 = property class="Camera"(reference=w325, error in=w324) -> (error out=w336:errorcluster, "Acquisition"=w335:refnum<k24>)  [unwired: 1 out]
        n207 = invoke class="Acquisition" method="HasStarted"(reference=w335, error in=w336) -> (reference out=w331:refnum<k24>, error out=w330:errorcluster, "HasStarted"=w329:i32, "bValue"=w334:bool)  [unwired: 2 in]
        n208 = invoke class="Acquisition" method="ToString"(reference=w331, error in=w330) -> (error out=w333:errorcluster, "ToString"=w332:string)  [unwired: 1 in, 1 out]
        n209 = call <instrlib>:"Error_Handling.vi"("Error Code"=w329, "Error String"=w332, "Error In"=w333) -> ("Error Out"=w328:errorcluster)  [unwired: 8 in]
        n210 = case shown="False" w334 {
          tunnel: [w339 w345] -> w326
          tunnel: w328 -> [w339 w344]
          tunnel: w325 -> [w338 w340]
          tunnel: [w338 w340] -> w327
          frame False {
          }
          frame True {
            # "Memory"
            n211 = property class="Camera"(reference=w340, error in=w344) -> (error out=w347:errorcluster, "Memory"=w348:refnum<k24>)  [unwired: 1 out]
            n212 = invoke class="Memory" method="GetActive"(reference=w348, error in=w347) -> (reference out=w354:refnum<k24>, error out=w353:errorcluster, "GetActive"=w355:i32, "s32MemId"=w346:i32)  [unwired: 2 in]
            n213 = invoke class="Memory" method="ToString"(reference=w354, error in=w353) -> (error out=w351:errorcluster, "ToString"=w352:string)  [unwired: 1 in, 1 out]
            n214 = call <instrlib>:"Error_Handling.vi"("Error Code"=w355, "Error String"=w352, "Error In"=w351) -> ("Error Out"=w356:errorcluster)  [unwired: 8 in]
            n215 = property class="Camera"(reference=w340, error in=w356) -> (error out=w350:errorcluster, "Memory"=w349:refnum<k24>)  [unwired: 1 out]
            n216 = invoke class="Memory" method="CopyToArray"(reference=w349, error in=w350, "s32MemId"=w346) -> (reference out=w359:refnum<k24>, error out=w360:errorcluster, "CopyToArray"=w361:i32, "u8Image"=w341:u8[])  [unwired: 2 in, 1 out]
            n217 = invoke class="Memory" method="ToString"(reference=w359, error in=w360) -> (error out=w357:errorcluster, "ToString"=w358:string)  [unwired: 1 in, 1 out]
            n218 = call <instrlib>:"Error_Handling.vi"("Error Code"=w361, "Error String"=w358, "Error In"=w357) -> ("Error Out"=w342:errorcluster)  [unwired: 8 in]
            n219 = call <instrlib>:"ArrayToImage.vi"("Error In"=w342, "InArray"=w341, ".NET (Reference)"=w340) -> ("Error Out"=w345:errorcluster, "Image"=→"Image second camera":picture)  [unwired: 7 in]
          }
        }
      }
      frame "Init camera" {
        w370 = 1 items=["IS_DONT_WAIT", "IS_WAIT"] ("Wait")
        w397 = 0 items=["RGB 32"=0, "RGB 24"=1, "Y8 Monochrom"=6] ("Mode")
        # "SubVI Example for \nGetDefault Timing"
        # "SubVI Example for \nMemory allocation"
        # "SubVI Example for \nTiming"
        # "SubVI Example for \nCamera Init"
        # "Pixelformat"
        n220 = control-ref of="Init Camera 2"() -> (w365:refnum<vi>)
        n221 = control-ref of="Exit Camera 2"() -> (w363:refnum<vi>)
        n222 = property class="Bool"(reference=w365, "Disabled"=u8 2 ("Deaktiviert")) -> ()  [unwired: 1 in, 2 out]
        n223 = property class="Bool"(reference=w363, "Disabled"=u8 0 ("Deaktiviert")) -> ()  [unwired: 1 in, 2 out]
        n224 = call <instrlib>:"SubVI_Example_CameraInit.vi"("Error In"=w389, "Camera ID"="Camera ID 3", "Init Camera Flag"=TRUE, ".NET (Reference)"=w390) -> ("Error Out"=w394:errorcluster, ".NET (Reference)"=w368:refnum<k24>)  [unwired: 6 in]
        n225 = property class="Camera"(reference=w368, error in=w394) -> (error out=w395:errorcluster, "PixelFormat"=w396:refnum<k24>)  [unwired: 1 out]
        n226 = invoke class="PixelFormat" method="Set"(reference=w396, error in=w395, "mode"=w397) -> (reference out=w392:refnum<k24>, error out=w386:errorcluster, "Set"=w391:i32)  [unwired: 1 in, 1 out]
        n227 = invoke class="PixelFormat" method="ToString"(reference=w392, error in=w386) -> (error out=w385:errorcluster, "ToString"=w393:string)  [unwired: 1 in, 1 out]
        n228 = call <instrlib>:"Error_Handling.vi"("Error Code"=w391, "Error String"=w393, "Error In"=w385) -> ("Error Out"=w382:errorcluster)  [unwired: 8 in]
        n229 = call <instrlib>:"SubVI_Example_GetDefault_Timing.vi"(".NET (Reference)"=w368, "Error In"=w382) -> ("Pixelclock"=w379:i32, "Exposure time"=w380:dbl, "Framerate"=w381:dbl, "Error Out"=w378:errorcluster)  [unwired: 10 in]
        n230 = call <instrlib>:"SubVI_Example_Timing.vi"(".NET (Reference)"=w368, "Pixelclock"=w379, "Exposure time"=w380, "Framerate"=w381, "Error In"=w378) -> ("Error Out"=w384:errorcluster)  [unwired: 7 in, 3 out]
        n231 = call <instrlib>:"SubVI_Example_MemoryAllocation.vi"(".NET (Reference)"=w368, "Error In"=w384) -> ("Serial Number"=→"Serial Number 2":string, "Error Out"=w367:errorcluster)  [unwired: 13 in, 3 out]
        n232 = property class="Camera"(reference=w368, error in=w367) -> (error out=w376:errorcluster, "Acquisition"=w377:refnum<k24>)  [unwired: 1 out]
        n233 = invoke class="Acquisition" method="Capture"(reference=w377, error in=w376, "param"=w370) -> (reference out=w372:refnum<k24>, error out=w373:errorcluster, "Capture"=w371:i32)  [unwired: 1 in, 1 out]
        n234 = invoke class="Acquisition" method="ToString"(reference=w372, error in=w373) -> (error out=w375:errorcluster, "ToString"=w374:string)  [unwired: 1 in, 1 out]
        n235 = call <instrlib>:"Error_Handling.vi"("Error Code"=w371, "Error String"=w374, "Error In"=w375) -> ("Error Out"=w369:errorcluster)  [unwired: 8 in]
      }
    }
    n236 = case shown="Default" w165 {
      tunnel: w156 -> [w408 w439 w504]
      tunnel: w155 -> [w409 w438 w503]
      tunnel: [w418 w441 w483] -> w158
      tunnel: [w419 w440 w484] -> w162
      tunnel: [TRUE FALSE FALSE] -> w160
      frame "Exit camera" {
        # "Close .Net Referenz"
        # "Is acquisition running?"
        # "Stop Acquisition"
        # "Close Camera"
        n237 = control-ref of="Init Camera"() -> (w403:refnum<vi>)
        n238 = control-ref of="Exit Camera"() -> (w402:refnum<vi>)
        n239 = property class="Camera"(reference=w408, error in=w409) -> (error out=w417:errorcluster, "Acquisition"=w416:refnum<k24>)  [unwired: 1 out]
        n240 = property class="Bool"(reference=w403, "Disabled"=u8 0 ("Deaktiviert")) -> ()  [unwired: 1 in, 2 out]
        n241 = property class="Bool"(reference=w402, "Disabled"=u8 2 ("Deaktiviert")) -> ()  [unwired: 1 in, 2 out]
        n242 = invoke class="Acquisition" method="HasStarted"(reference=w416, error in=w417) -> (reference out=w410:refnum<k24>, error out=w413:errorcluster, "bValue"=w415:bool)  [unwired: 2 in, 1 out]
        n243 = invoke class="Acquisition" method="ToString"(reference=w410, error in=w413) -> (error out=w412:errorcluster, "ToString"=w411:string)  [unwired: 1 in, 1 out]
        n244 = call <instrlib>:"Error_Handling.vi"("Error String"=w411, "Error In"=w412) -> ("Error Out"=w414:errorcluster)  [unwired: 9 in]
        n245 = case shown="True" w415 {
          tunnel: [w427 w436] -> w406
          tunnel: w414 -> [w427 w437]
          tunnel: w408 -> [w426 w428]
          tunnel: [w426 w428] -> w407
          frame False {
          }
          frame True {
            n246 = property class="Camera"(reference=w428, error in=w437) -> (error out=w432:errorcluster, "Acquisition"=w433:refnum<k24>)  [unwired: 1 out]
            n247 = invoke class="Acquisition" method="Stop"(reference=w433, error in=w432) -> (reference out=w430:refnum<k24>, error out=w431:errorcluster, "Stop"=w429:i32)  [unwired: 1 in]
            n248 = invoke class="Acquisition" method="ToString"(reference=w430, error in=w431) -> (error out=w435:errorcluster, "ToString"=w434:string)  [unwired: 1 in, 1 out]
            n249 = call <instrlib>:"Error_Handling.vi"("Error Code"=w429, "Error String"=w434, "Error In"=w435) -> ("Error Out"=w436:errorcluster)  [unwired: 8 in]
          }
        }
        n250 = invoke class="Camera" method="Exit"(reference=w407, error in=w406) -> (reference out=w418:refnum<k24>, error out=w422:errorcluster, "Exit"=w421:i32)  [unwired: 1 in]
        n251 = invoke class="Camera" method="ToString"(reference=w418, error in=w422) -> (error out=w423:errorcluster, "ToString"=w424:string)  [unwired: 1 in, 1 out]
        n252 = call <instrlib>:"Error_Handling.vi"("Error Code"=w421, "Error String"=w424, "Error In"=w423) -> ("Error Out"=w420:errorcluster)  [unwired: 8 in]
        n253 = Close Reference ("Close Referenz")(reference=w418, error in (no error)=w420) -> (error out=w419:errorcluster)
      }
      frame Default {
        # "Has acquisition started?"
        n254 = property class="Camera"(reference=w439, error in=w438) -> (error out=w450:errorcluster, "Acquisition"=w449:refnum<k24>)  [unwired: 1 out]
        n255 = invoke class="Acquisition" method="HasStarted"(reference=w449, error in=w450) -> (reference out=w445:refnum<k24>, error out=w444:errorcluster, "HasStarted"=w443:i32, "bValue"=w448:bool)  [unwired: 2 in]
        n256 = invoke class="Acquisition" method="ToString"(reference=w445, error in=w444) -> (error out=w447:errorcluster, "ToString"=w446:string)  [unwired: 1 in, 1 out]
        n257 = call <instrlib>:"Error_Handling.vi"("Error Code"=w443, "Error String"=w446, "Error In"=w447) -> ("Error Out"=w442:errorcluster)  [unwired: 8 in]
        n258 = case shown="True" w448 {
          tunnel: [w453 w459] -> w440
          tunnel: w442 -> [w453 w458]
          tunnel: w439 -> [w452 w456]
          tunnel: [w452 w456] -> w441
          frame False {
            # "Show Image"
          }
          frame True {
            # "Memory"
            n259 = property class="Camera"(reference=w456, error in=w458) -> (error out=w461:errorcluster, "Memory"=w462:refnum<k24>)  [unwired: 1 out]
            n260 = invoke class="Memory" method="GetActive"(reference=w462, error in=w461) -> (reference out=w468:refnum<k24>, error out=w467:errorcluster, "GetActive"=w469:i32, "s32MemId"=w460:i32)  [unwired: 2 in]
            n261 = invoke class="Memory" method="ToString"(reference=w468, error in=w467) -> (error out=w465:errorcluster, "ToString"=w466:string)  [unwired: 1 in, 1 out]
            n262 = call <instrlib>:"Error_Handling.vi"("Error Code"=w469, "Error String"=w466, "Error In"=w465) -> ("Error Out"=w470:errorcluster)  [unwired: 8 in]
            n263 = property class="Camera"(reference=w456, error in=w470) -> (error out=w464:errorcluster, "Memory"=w463:refnum<k24>)  [unwired: 1 out]
            n264 = invoke class="Memory" method="CopyToArray"(reference=w463, error in=w464, "s32MemId"=w460) -> (reference out=w473:refnum<k24>, error out=w474:errorcluster, "CopyToArray"=w475:i32, "u8Image"=w455:u8[])  [unwired: 2 in, 1 out]
            n265 = invoke class="Memory" method="ToString"(reference=w473, error in=w474) -> (error out=w471:errorcluster, "ToString"=w472:string)  [unwired: 1 in, 1 out]
            n266 = call <instrlib>:"Error_Handling.vi"("Error Code"=w475, "Error String"=w472, "Error In"=w471) -> ("Error Out"=w457:errorcluster)  [unwired: 8 in]
            n267 = call <instrlib>:"ArrayToImage.vi"("Error In"=w457, "InArray"=w455, ".NET (Reference)"=w456) -> ("Error Out"=w459:errorcluster, "Image"=→"Image first camera":picture)  [unwired: 7 in]
          }
        }
      }
      frame "Init camera" {
        w485 = 1 items=["IS_DONT_WAIT", "IS_WAIT"] ("Wait")
        w511 = 0 items=["RGB 32"=0, "RGB 24"=1, "Y8 Monochrom"=6] ("Mode")
        # "SubVI Example for \nGetDefault Timing"
        # "SubVI Example for \nMemory allocation"
        # "SubVI Example for \nTiming"
        # "SubVI Example for \nCamera Init"
        # "Pixelformat"
        n268 = control-ref of="Init Camera"() -> (w479:refnum<vi>)
        n269 = control-ref of="Exit Camera"() -> (w477:refnum<vi>)
        n270 = call <instrlib>:"SubVI_Example_CameraInit.vi"("Error In"=w503, "Camera ID"="Camera ID 1", "Init Camera Flag"=TRUE, ".NET (Reference)"=w504) -> ("Error Out"=w508:errorcluster, ".NET (Reference)"=w483:refnum<k24>)  [unwired: 6 in]
        n271 = property class="Bool"(reference=w479, "Disabled"=u8 2 ("Deaktiviert")) -> ()  [unwired: 1 in, 2 out]
        n272 = property class="Bool"(reference=w477, "Disabled"=u8 0 ("Deaktiviert")) -> ()  [unwired: 1 in, 2 out]
        n273 = property class="Camera"(reference=w483, error in=w508) -> (error out=w509:errorcluster, "PixelFormat"=w510:refnum<k24>)  [unwired: 1 out]
        n274 = invoke class="PixelFormat" method="Set"(reference=w510, error in=w509, "mode"=w511) -> (reference out=w506:refnum<k24>, error out=w500:errorcluster, "Set"=w505:i32)  [unwired: 1 in, 1 out]
        n275 = invoke class="PixelFormat" method="ToString"(reference=w506, error in=w500) -> (error out=w499:errorcluster, "ToString"=w507:string)  [unwired: 1 in, 1 out]
        n276 = call <instrlib>:"Error_Handling.vi"("Error Code"=w505, "Error String"=w507, "Error In"=w499) -> ("Error Out"=w496:errorcluster)  [unwired: 8 in]
        n277 = call <instrlib>:"SubVI_Example_GetDefault_Timing.vi"(".NET (Reference)"=w483, "Error In"=w496) -> ("Pixelclock"=w493:i32, "Exposure time"=w494:dbl, "Framerate"=w495:dbl, "Error Out"=w481:errorcluster)  [unwired: 10 in]
        n278 = call <instrlib>:"SubVI_Example_Timing.vi"(".NET (Reference)"=w483, "Pixelclock"=w493, "Exposure time"=w494, "Framerate"=w495, "Error In"=w481) -> ("Error Out"=w498:errorcluster)  [unwired: 7 in, 3 out]
        n279 = call <instrlib>:"SubVI_Example_MemoryAllocation.vi"(".NET (Reference)"=w483, "Error In"=w498) -> ("Serial Number"=→"Serial Number 1":string, "Error Out"=w482:errorcluster)  [unwired: 13 in, 3 out]
        n280 = property class="Camera"(reference=w483, error in=w482) -> (error out=w491:errorcluster, "Acquisition"=w492:refnum<k24>)  [unwired: 1 out]
        n281 = invoke class="Acquisition" method="Capture"(reference=w492, error in=w491, "param"=w485) -> (reference out=w487:refnum<k24>, error out=w488:errorcluster, "Capture"=w486:i32)  [unwired: 1 in, 1 out]
        n282 = invoke class="Acquisition" method="ToString"(reference=w487, error in=w488) -> (error out=w490:errorcluster, "ToString"=w489:string)  [unwired: 1 in, 1 out]
        n283 = call <instrlib>:"Error_Handling.vi"("Error Code"=w486, "Error String"=w489, "Error In"=w490) -> ("Error Out"=w484:errorcluster)  [unwired: 8 in]
      }
    }
    n284 = case shown="False" "steps /\n continuous \ntoggle" {
      tunnel: w129 -> [w186 w262]
      tunnel: w128 -> [w185 w261]
      tunnel: [w204 w268] -> w127
      tunnel: [w177 w274] -> w117
      tunnel: "up a1" -> [w203 w270]
      tunnel: "down a1" -> [w201 w269]
      tunnel: "up all" -> [w184 w257]
      tunnel: "down all" -> [w183 w258]
      tunnel: "down a3" -> [w191 w266]
      tunnel: "up a3" -> [w192 w265]
      tunnel: "down a2" -> [w189 w260]
      tunnel: "up a2" -> [w190 w259]
      tunnel: w122 -> [_ w272]
      tunnel: [_ w273] -> w126
      tunnel: [_ w253] -> w125
      tunnel: w121 -> [_ w250]
      tunnel: [_ w251] -> w123
      tunnel: w119 -> [_ w248]
      tunnel: [_ w252] -> w124
      tunnel: w120 -> [_ w249]
      frame False {
        n285 = flat-sequence {
          tunnel: w186 -> [w219]
          tunnel: w185 -> [w222]
          tunnel: w192 -> [w217]
          tunnel: "a3" ("Combo Box") -> [w215]
          tunnel: "Step size" -> [w218]
          tunnel: w191 -> [w216]
          tunnel: [w221] -> w195
          tunnel: [w220] -> w194
          tunnel: [w224] -> _
          tunnel: [w225] -> w179
          tunnel: w195 -> [w225]
          tunnel: w194 -> [w224]
          frame #0 {
            n286 = call "Picomotor step single.vi"("Step size"=w218, "Combo Box"=w215, "error in (no error)"=w222, "down a1"=w216, "up a1"=w217, "VISA Refnum in"=w219) -> ("error out"=w221:errorcluster, "VISA Refnum out"=w220:refnum<visa-resource-name>)  [unwired: 4 in]
          }
          frame #1 {
            n287 = Wait (ms)(milliseconds to wait=u32 100) -> ()  [unwired: 1 out]
          }
        }
        n288 = flat-sequence {
          tunnel: w186 -> [w241]
          tunnel: w185 -> [w244]
          tunnel: w203 -> [w239]
          tunnel: "a1" ("Combo Box") -> [w237]
          tunnel: "Step size" -> [w240]
          tunnel: w201 -> [w238]
          tunnel: [w243] -> w200
          tunnel: [w242] -> w199
          tunnel: [w246] -> w204
          tunnel: [w247] -> w181
          tunnel: w200 -> [w247]
          tunnel: w199 -> [w246]
          frame #0 {
            n289 = call "Picomotor step single.vi"("Step size"=w240, "Combo Box"=w237, "error in (no error)"=w244, "down a1"=w238, "up a1"=w239, "VISA Refnum in"=w241) -> ("error out"=w243:errorcluster, "VISA Refnum out"=w242:refnum<visa-resource-name>)  [unwired: 4 in]
          }
          frame #1 {
            n290 = Wait (ms)(milliseconds to wait=u32 100) -> ()  [unwired: 1 out]
          }
        }
        n291 = flat-sequence {
          tunnel: w186 -> [w230]
          tunnel: w185 -> [w233]
          tunnel: w190 -> [w228]
          tunnel: "a2" ("Combo Box") -> [w226]
          tunnel: "Step size" -> [w229]
          tunnel: w189 -> [w227]
          tunnel: [w232] -> w198
          tunnel: [w231] -> w197
          tunnel: [w235] -> _
          tunnel: [w236] -> w180
          tunnel: w198 -> [w236]
          tunnel: w197 -> [w235]
          frame #0 {
            n292 = call "Picomotor step single.vi"("Step size"=w229, "Combo Box"=w226, "error in (no error)"=w233, "down a1"=w227, "up a1"=w228, "VISA Refnum in"=w230) -> ("error out"=w232:errorcluster, "VISA Refnum out"=w231:refnum<visa-resource-name>)  [unwired: 4 in]
          }
          frame #1 {
            n293 = Wait (ms)(milliseconds to wait=u32 100) -> ()  [unwired: 1 out]
          }
        }
        n294 = flat-sequence {
          tunnel: [w211] -> w188
          tunnel: [w210] -> w187
          tunnel: w186 -> [w209]
          tunnel: w185 -> [w208]
          tunnel: w184 -> [w207]
          tunnel: w183 -> [w206]
          tunnel: "Step size" -> [w205]
          tunnel: [w213] -> _
          tunnel: [w214] -> w178
          tunnel: w188 -> [w214]
          tunnel: w187 -> [w213]
          frame #0 {
            n295 = call "Picomotor step multi.vi"("Step size"=w205, "error in (no error)"=w208, "down a1"=w206, "up a1"=w207, "VISA Refnum in"=w209) -> ("error out"=w211:errorcluster, "VISA Refnum out"=w210:refnum<visa-resource-name>)  [unwired: 5 in]
          }
          frame #1 {
            n296 = Wait (ms)(milliseconds to wait=u32 100) -> ()  [unwired: 1 out]
          }
        }
        n297 = Merge Errors(w181, w180, w179, w178) -> (w177:errorcluster)
      }
      frame True {
        n298 = call "Picomotor single motor continuous.vi"("Enum"=w272, "Combo Box"="a1", "error in (no error)"=w261, "down"=w269, "up"=w270, "VISA Refnum in"=w262) -> ("error out"=w267:errorcluster, "Numeric"=w273:i32, "VISA Refnum out"=w268:refnum<visa-resource-name>)  [unwired: 3 in]
        n299 = call "Picomotor single motor continuous.vi"("Enum"=w249, "Combo Box"="a3", "error in (no error)"=w261, "down"=w266, "up"=w265, "VISA Refnum in"=w262) -> ("error out"=w255:errorcluster, "Numeric"=w252:i32)  [unwired: 3 in, 1 out]
        n300 = call "Picomotor single motor continuous.vi"("Enum"=w250, "Combo Box"="a2", "error in (no error)"=w261, "down"=w260, "up"=w259, "VISA Refnum in"=w262) -> ("error out"=w256:errorcluster, "Numeric"=w253:i32)  [unwired: 3 in, 1 out]
        n301 = call "Picomotor all motors continuous.vi"("Enum"=w248, "error in (no error)"=w261, "down"=w258, "up"=w257, "VISA Refnum in"=w262) -> ("error out"=w254:errorcluster, "Numeric"=w251:i32)  [unwired: 4 in, 1 out]
        n302 = Merge Errors(w267, w256, w255, w254) -> (w274:errorcluster)
      }
    }
    n303 = call <instrlib>:"SubVI_Example_SyncEventLoop.vi"("Error In"=w149, "use sync"=w147, ".NET (Reference)"=w145) -> ("Error Out"=w144:errorcluster, "Synchronize (ms)"=w148:dbl)  [unwired: 7 in]
    "Error Camera 2" <- w144
    n304 = call <instrlib>:"SubVI_Example_SyncEventLoop.vi"("Error In"=w162, "use sync"=w160, ".NET (Reference)"=w158) -> ("Error Out"=w157:errorcluster, "Synchronize (ms)"=w161:dbl)  [unwired: 7 in]
    "Error Camera 1" <- w157
    n305 = Wait Until Next ms Multiple(millisecond multiple=w161) -> ()  [unwired: 1 out]
    n306 = Wait Until Next ms Multiple(millisecond multiple=w148) -> ()  [unwired: 1 out]
    n307 = case shown="False" "stop" {
      tunnel: w127 -> [w277 w282]
      tunnel: w117 -> [w276 w281]
      tunnel: [w277 w280] -> w116
      tunnel: [w276 w279] -> w118
      tunnel: [w275 w278] -> w140
      tunnel: "stop" -> [w275 w278]
      frame False {
      }
      frame True {
        n308 = call "Picomotor Write.vi"("error in (no error)"=w281, "String 3"="sto", "VISA Refnum in"=w282) -> ("error out"=w279:errorcluster, "VISA Refnum out"=w280:refnum<visa-resource-name>)  [unwired: 6 in, 1 out]
      }
    }
    n309 = Merge Errors(w118, w117) -> (w141:errorcluster)
  }
  n310 = VISA Close(VISA resource name=w5, error in (no error)=w6) -> (error out=→"error":errorcluster)
